vi "Get Enclave.vi"(11 "Writer in":refnum<class "Writer.lvclass">) -> (2 "Enclave":refnum<class "Enclave.lvclass">)   [LabVIEW 2022 SP3, in "Enclave.lvlib" / "Writer.lvclass"]
uses:
  Writer.lvclass
  Writer.lvclass/Writer.ctl
  Enclave/Enclave.lvclass
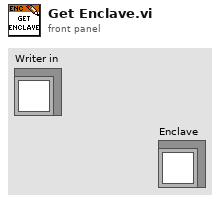
[diagram p1: front panel]
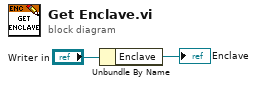
[diagram p0: block diagram]
diagram:
  n1 = Unbundle By Name("Writer in") -> ("Enclave"=→"Enclave":refnum<class "Enclave.lvclass">)
